vi "name_file_by_time_stamp.vi"(11 "Folder to save file to":path=path "C:/Users/LAV-UFSC-2023/Documents/LAV-TCC/Dados-Experimentos/Dados-Bancada-LABVIEW") -> (3 "New file path":path)   [LabVIEW 2022 SP3]
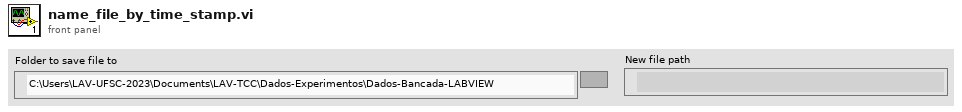
[diagram p1: front panel]
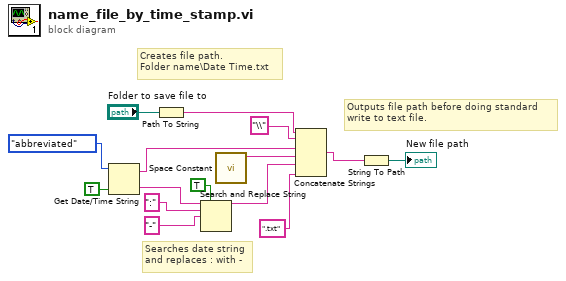
[diagram p0: block diagram]
diagram:
  # "Searches date string\nand replaces : with -"
  # "Creates file path.\nFolder name\\Date Time.txt"
  # "Outputs file path before doing standard\nwrite to text file."
  n1 = Get Date/Time String(date format (0)=enum16{"short", "long", "abbreviated"}."abbreviated", want seconds? (F)=TRUE) -> (date string=w2:string, time string=w13:string)  [unwired: 1 in]
  n2 = Path To String(path="Folder to save file to") -> (string=w5:string)
  n3 = Search and Replace String(replace all?=TRUE ("replace all? (F)"), input string=w13, search string=":" ("replace string (\"\")"), replace string="-" ("replace string (\"\")")) -> (result string=w3:string)  [unwired: 4 in, 3 out]
  n4 = call <vilib>:"Space Constant.vi"() -> ("String"=w9:string)
  n5 = Concatenate Strings(w5, "\\" ("string"), w2, w9, w3, ".txt" ("string")) -> (w7:string)
  n6 = String To Path(string=w7) -> (path=→"New file path":path)
